vi "LowerLevelSortArrays.vi"(0 "Sorted Array in":string[](array[string]), 1 "DIM-Double-Array":refnum<vi>[](array[refnum]), 2 "DIM-Double":refnum<vi>[](array[refnum]), 3 "DigitalNumeric":refnum<vi>[](array[refnum]), 4 "Boolean":refnum<vi>[](array[refnum]), 5 "DIM-Short":refnum<vi>[](array[refnum]), 6 "Boolean(Strict)":refnum<vi>[](array[refnum]), 7 "Unsorted Array in":string[](array[string]), 8 "Index":i32, 10 "Type":T1(ring)) -> (21 "DIM-Double-Array (sorted)":refnum<vi>[](array[refnum]), 22 "DIM-Double (sorted)":refnum<vi>[](array[refnum]), 23 "DigitalNumeric (sorted)":refnum<vi>[](array[refnum]), 24 "Boolean (sorted)":refnum<vi>[](array[refnum]), 25 "DIM-Short(sorted)":refnum<vi>[](array[refnum]), 26 "Boolean (Strict) (sorted)":refnum<vi>[](array[refnum]), 27 "Sorted Array out":string[](array[string]))   [LabVIEW 2014, in "Panels.lvlib"]
uses:
  Panels.lvlib
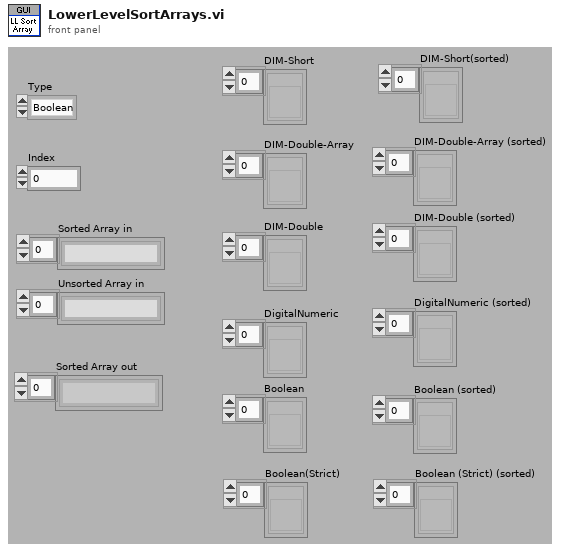
[diagram p1: front panel]
types:
  T1 = enum16{"Boolean", "DigitalNumeric", "DIM-Double", "DIM-Double-Array", "DIM-Short", "Boolean (Strict)"}
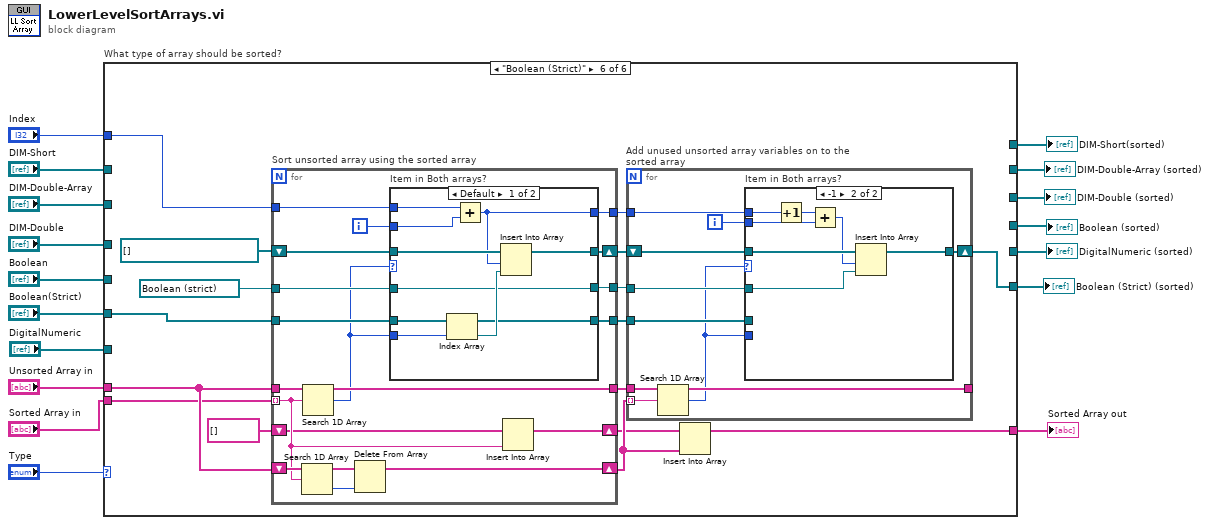
[diagram p0: block diagram]
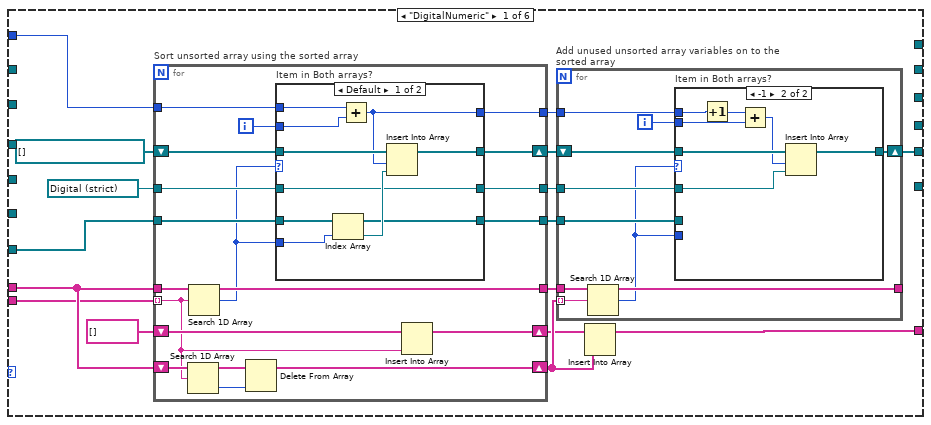
[diagram p2: hidden frame]
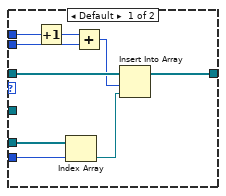
[diagram p3: hidden frame]
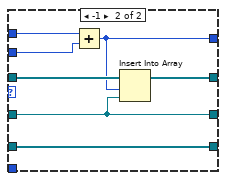
[diagram p4: hidden frame]
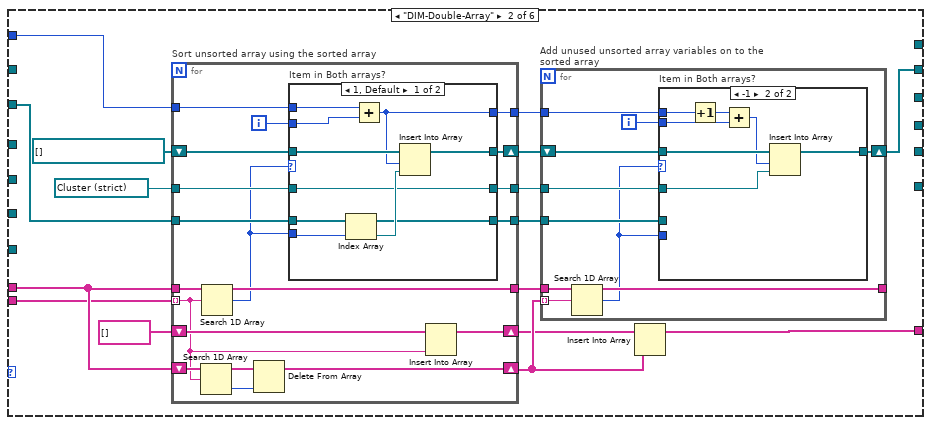
[diagram p5: hidden frame]
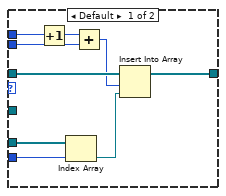
[diagram p6: hidden frame]
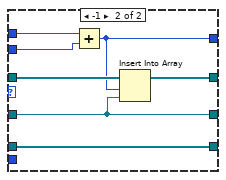
[diagram p7: hidden frame]
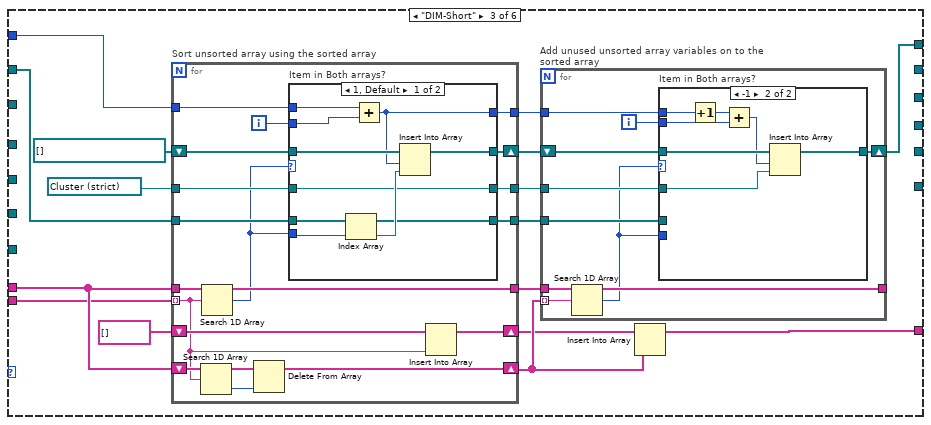
[diagram p8: hidden frame]
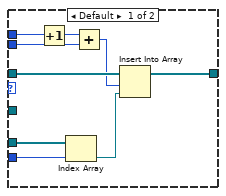
[diagram p9: hidden frame]
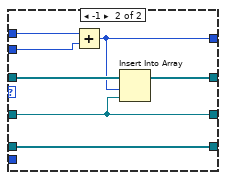
[diagram p10: hidden frame]
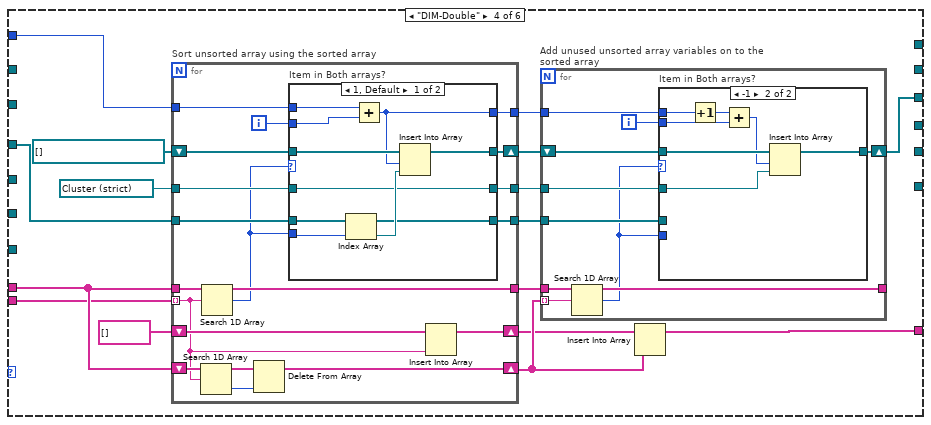
[diagram p11: hidden frame]
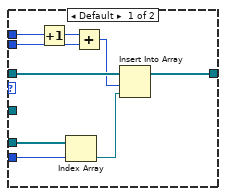
[diagram p12: hidden frame]
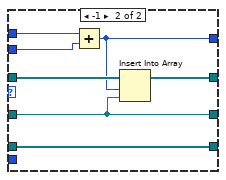
[diagram p13: hidden frame]
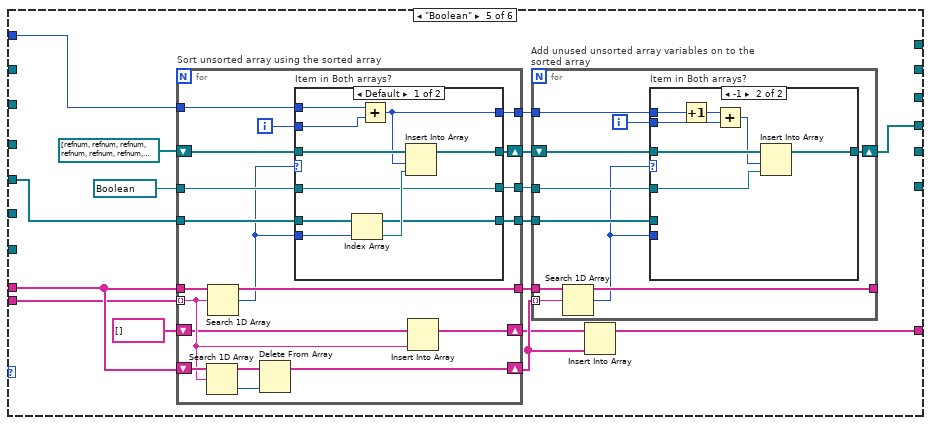
[diagram p14: hidden frame]
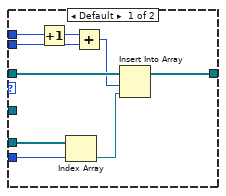
[diagram p15: hidden frame]
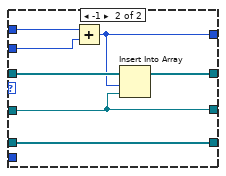
[diagram p16: hidden frame]
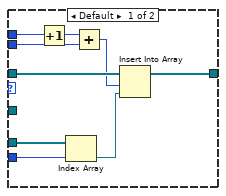
[diagram p17: hidden frame]
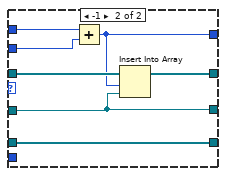
[diagram p18: hidden frame]
diagram:
  n1 = case "What type of array should be sorted?" shown="\"Boolean (Strict)\"" "Type" {
    tunnel: "DigitalNumeric" -> [w32 _ _ _ _ _]
    tunnel: "Unsorted Array in" -> [w31 w105 w179 w250 w324 w400]
    tunnel: "Sorted Array in" -> [w27 w104 w178 w249 w323 w399]
    tunnel: "Index" -> [w30 w107 w181 w255 w329 w403]
    tunnel: "Boolean" -> [_ _ _ _ w326 _]
    tunnel: "DIM-Double" -> [_ _ _ w252 _ _]
    tunnel: [_ _ _ w244 _ _] -> w9
    tunnel: [w28 w106 w180 w251 w325 w401] -> w10
    tunnel: [_ _ _ _ w316 _] -> w8
    tunnel: [w20 _ _ _ _ _] -> w7
    tunnel: "DIM-Double-Array" -> [_ w95 _ _ _ _]
    tunnel: [_ w92 _ _ _ _] -> w5
    tunnel: "DIM-Short" -> [_ _ w169 _ _ _]
    tunnel: [_ _ w168 _ _ _] -> w3
    tunnel: "Boolean(Strict)" -> [_ _ _ _ _ w389]
    tunnel: [_ _ _ _ _ w388] -> w1
    frame "DigitalNumeric" {
      n2 = for "Sort unsorted array using the sorted array" {
        tunnel: w27 -> [w59] mode=indexing
        tunnel: w31 -> [w71]
        tunnel: w32 -> [w72]
        shift-right: [w74] -> w25
        shift-left: refnum<vi>[] [] ("FPIndicator") -> [w75]
        tunnel: [w67] -> w26
        shift-right: [w73] -> w21
        shift-left: w31 -> [w70]
        tunnel: [w71] -> w22
        tunnel: w30 -> [w69]
        tunnel: refnum<vi> refnum ("Q90DefMain_Mon") -> [w66]
        tunnel: [w64] -> w24
        tunnel: [w63] -> w23
        shift-right: [w60] -> w18
        shift-left: string[] [] -> [w61]
        i -> [w68]
        n3 = Search 1D Array(1D array=w70, element=w59) -> (index of element=w65:i32)  [unwired: 1 in]
        n4 = Search 1D Array(1D array=w71, element=w59) -> (index of element=w62:i32)  [unwired: 1 in]
        n5 = Delete From Array(array=w70, index=w65) -> (array with subset deleted=w73:string[])  [unwired: 1 in, 1 out]
        n6 = case "Item in Both arrays?" shown="Default" w62 {
          tunnel: w75 -> [w84 w91]
          tunnel: [w82 w90] -> w74
          tunnel: w72 -> [w76 w85]
          tunnel: w62 -> [w81 _]
          tunnel: w69 -> [w78 w87]
          tunnel: w68 -> [w80 w89]
          tunnel: [w79 w88] -> w67
          tunnel: w66 -> [w77 w86]
          tunnel: [w77 w86] -> w64
          tunnel: [w76 w85] -> w63
          frame Default {
            n7 = Index Array(array=w76, index=w81) -> (element=w83:refnum<vi>)
            n8 = Add(x=w78, y=w80) -> (x+y=w79:i32)
            n9 = Insert Into Array(array=w84, index=w79, new element=w83) -> (w82:refnum<vi>[])
          }
          frame -1 {
            n10 = Add(x=w87, y=w89) -> (x+y=w88:i32)
            n11 = Insert Into Array(array=w91, index=w88, new element=w86) -> (w90:refnum<vi>[])
          }
        }
        n12 = Insert Into Array(array=w61, new element=w59) -> (w60:string[])  [unwired: 1 in]
      }
      n13 = for "Add unused unsorted array variables on to the sorted array" {
        tunnel: w21 -> [w34] mode=indexing
        tunnel: w22 -> [w39]
        tunnel: w23 -> [w40]
        shift-right: [w41] -> w20
        shift-left: w25 -> [w42]
        tunnel: [w39] -> _
        tunnel: w26 -> [w38]
        tunnel: w24 -> [w36]
        i -> [w37]
        n14 = Search 1D Array(1D array=w39, element=w34) -> (index of element=w35:i32)  [unwired: 1 in]
        n15 = case "Item in Both arrays?" shown="-1" w35 {
          tunnel: w42 -> [w51 w58]
          tunnel: [w49 w57] -> w41
          tunnel: w40 -> [w48 _]
          tunnel: w35 -> [w47 _]
          tunnel: w38 -> [w43 w52]
          tunnel: w37 -> [w46 w56]
          tunnel: w36 -> [_ w54]
          frame Default {
            n16 = Increment(x=w43) -> (x+1=w44:i32)
            n17 = Index Array(array=w48, index=w47) -> (element=w50:refnum<vi>)
            n18 = Add(x=w44, y=w46) -> (x+y=w45:i32)
            n19 = Insert Into Array(array=w51, index=w45, new element=w50) -> (w49:refnum<vi>[])
          }
          frame -1 {
            n20 = Increment(x=w52) -> (x+1=w53:i32)
            n21 = Add(x=w53, y=w56) -> (x+y=w55:i32)
            n22 = Insert Into Array(array=w58, index=w55, new element=w54) -> (w57:refnum<vi>[])
          }
        }
      }
      n23 = Insert Into Array(array=w18, new element=w21) -> (w28:string[])  [unwired: 1 in]
    }
    frame "DIM-Double-Array" {
      n24 = for "Sort unsorted array using the sorted array" {
        tunnel: w104 -> [w133] mode=indexing
        tunnel: w105 -> [w145]
        tunnel: w95 -> [w146]
        shift-right: [w148] -> w102
        shift-left: refnum<vi>[] [] ("appended array") -> [w149]
        tunnel: [w140] -> w103
        shift-right: [w147] -> w100
        shift-left: w105 -> [w143]
        tunnel: [w145] -> w101
        tunnel: w107 -> [w142]
        tunnel: refnum<vi> refnum ("GasCellBase_SetData") -> [w139]
        tunnel: [w138] -> w99
        tunnel: [w137] -> w98
        shift-right: [w135] -> w96
        shift-left: string[] [] -> [w134]
        i -> [w141]
        n25 = Search 1D Array(1D array=w143, element=w133) -> (index of element=w144:i32)  [unwired: 1 in]
        n26 = Search 1D Array(1D array=w145, element=w133) -> (index of element=w136:i32)  [unwired: 1 in]
        n27 = Delete From Array(array=w143, index=w144) -> (array with subset deleted=w147:string[])  [unwired: 1 in, 1 out]
        n28 = case "Item in Both arrays?" shown="1, Default" w136 {
          tunnel: w149 -> [w158 w165]
          tunnel: [w156 w164] -> w148
          tunnel: w146 -> [w150 w159]
          tunnel: w136 -> [w155 _]
          tunnel: w142 -> [w152 w161]
          tunnel: w141 -> [w154 w163]
          tunnel: [w153 w162] -> w140
          tunnel: w139 -> [w151 w160]
          tunnel: [w151 w160] -> w138
          tunnel: [w150 w159] -> w137
          frame 1, Default {
            n29 = Index Array(array=w150, index=w155) -> (element=w157:refnum<vi>)
            n30 = Add(x=w152, y=w154) -> (x+y=w153:i32)
            n31 = Insert Into Array(array=w158, index=w153, new element=w157) -> (w156:refnum<vi>[])
          }
          frame -1 {
            n32 = Add(x=w161, y=w163) -> (x+y=w162:i32)
            n33 = Insert Into Array(array=w165, index=w162, new element=w160) -> (w164:refnum<vi>[])
          }
        }
        n34 = Insert Into Array(array=w134, new element=w133) -> (w135:string[])  [unwired: 1 in]
      }
      n35 = for "Add unused unsorted array variables on to the sorted array" {
        tunnel: w100 -> [w108] mode=indexing
        tunnel: w101 -> [w113]
        tunnel: w98 -> [w114]
        shift-right: [w115] -> w92
        shift-left: w102 -> [w116]
        tunnel: [w113] -> _
        tunnel: w103 -> [w112]
        tunnel: w99 -> [w110]
        i -> [w111]
        n36 = Search 1D Array(1D array=w113, element=w108) -> (index of element=w109:i32)  [unwired: 1 in]
        n37 = case "Item in Both arrays?" shown="-1" w109 {
          tunnel: w116 -> [w125 w132]
          tunnel: [w123 w131] -> w115
          tunnel: w114 -> [w122 _]
          tunnel: w109 -> [w121 _]
          tunnel: w112 -> [w117 w126]
          tunnel: w111 -> [w120 w130]
          tunnel: w110 -> [_ w128]
          frame Default {
            n38 = Increment(x=w117) -> (x+1=w118:i32)
            n39 = Index Array(array=w122, index=w121) -> (element=w124:refnum<vi>)
            n40 = Add(x=w118, y=w120) -> (x+y=w119:i32)
            n41 = Insert Into Array(array=w125, index=w119, new element=w124) -> (w123:refnum<vi>[])
          }
          frame -1 {
            n42 = Increment(x=w126) -> (x+1=w127:i32)
            n43 = Add(x=w127, y=w130) -> (x+y=w129:i32)
            n44 = Insert Into Array(array=w132, index=w129, new element=w128) -> (w131:refnum<vi>[])
          }
        }
      }
      n45 = Insert Into Array(array=w96, new element=w100) -> (w106:string[])  [unwired: 1 in]
    }
    frame "DIM-Short" {
      n46 = for "Sort unsorted array using the sorted array" {
        tunnel: w178 -> [w207] mode=indexing
        tunnel: w179 -> [w219]
        tunnel: w169 -> [w220]
        shift-right: [w222] -> w176
        shift-left: refnum<vi>[] [] ("DIM-Short") -> [w223]
        tunnel: [w214] -> w177
        shift-right: [w221] -> w174
        shift-left: w179 -> [w217]
        tunnel: [w219] -> w175
        tunnel: w181 -> [w216]
        tunnel: refnum<vi> refnum ("BOB6FVout_MonData") -> [w213]
        tunnel: [w212] -> w173
        tunnel: [w211] -> w172
        shift-right: [w209] -> w170
        shift-left: string[] [] -> [w208]
        i -> [w215]
        n47 = Search 1D Array(1D array=w217, element=w207) -> (index of element=w218:i32)  [unwired: 1 in]
        n48 = Search 1D Array(1D array=w219, element=w207) -> (index of element=w210:i32)  [unwired: 1 in]
        n49 = Delete From Array(array=w217, index=w218) -> (array with subset deleted=w221:string[])  [unwired: 1 in, 1 out]
        n50 = case "Item in Both arrays?" shown="1, Default" w210 {
          tunnel: w223 -> [w232 w239]
          tunnel: [w230 w238] -> w222
          tunnel: w220 -> [w224 w233]
          tunnel: w210 -> [w229 _]
          tunnel: w216 -> [w226 w235]
          tunnel: w215 -> [w228 w237]
          tunnel: [w227 w236] -> w214
          tunnel: w213 -> [w225 w234]
          tunnel: [w225 w234] -> w212
          tunnel: [w224 w233] -> w211
          frame 1, Default {
            n51 = Index Array(array=w224, index=w229) -> (element=w231:refnum<vi>)
            n52 = Add(x=w226, y=w228) -> (x+y=w227:i32)
            n53 = Insert Into Array(array=w232, index=w227, new element=w231) -> (w230:refnum<vi>[])
          }
          frame -1 {
            n54 = Add(x=w235, y=w237) -> (x+y=w236:i32)
            n55 = Insert Into Array(array=w239, index=w236, new element=w234) -> (w238:refnum<vi>[])
          }
        }
        n56 = Insert Into Array(array=w208, new element=w207) -> (w209:string[])  [unwired: 1 in]
      }
      n57 = for "Add unused unsorted array variables on to the sorted array" {
        tunnel: w174 -> [w182] mode=indexing
        tunnel: w175 -> [w187]
        tunnel: w172 -> [w188]
        shift-right: [w189] -> w168
        shift-left: w176 -> [w190]
        tunnel: [w187] -> _
        tunnel: w177 -> [w186]
        tunnel: w173 -> [w184]
        i -> [w185]
        n58 = Search 1D Array(1D array=w187, element=w182) -> (index of element=w183:i32)  [unwired: 1 in]
        n59 = case "Item in Both arrays?" shown="-1" w183 {
          tunnel: w190 -> [w199 w206]
          tunnel: [w197 w205] -> w189
          tunnel: w188 -> [w196 _]
          tunnel: w183 -> [w195 _]
          tunnel: w186 -> [w191 w200]
          tunnel: w185 -> [w194 w204]
          tunnel: w184 -> [_ w202]
          frame Default {
            n60 = Increment(x=w191) -> (x+1=w192:i32)
            n61 = Index Array(array=w196, index=w195) -> (element=w198:refnum<vi>)
            n62 = Add(x=w192, y=w194) -> (x+y=w193:i32)
            n63 = Insert Into Array(array=w199, index=w193, new element=w198) -> (w197:refnum<vi>[])
          }
          frame -1 {
            n64 = Increment(x=w200) -> (x+1=w201:i32)
            n65 = Add(x=w201, y=w204) -> (x+y=w203:i32)
            n66 = Insert Into Array(array=w206, index=w203, new element=w202) -> (w205:refnum<vi>[])
          }
        }
      }
      n67 = Insert Into Array(array=w170, new element=w174) -> (w180:string[])  [unwired: 1 in]
    }
    frame "DIM-Double" {
      n68 = for "Sort unsorted array using the sorted array" {
        tunnel: w249 -> [w281] mode=indexing
        tunnel: w250 -> [w293]
        tunnel: w252 -> [w294]
        shift-right: [w296] -> w247
        shift-left: refnum<vi>[] [] ("DIMControlMon") -> [w297]
        tunnel: [w288] -> w248
        shift-right: [w295] -> w245
        shift-left: w250 -> [w291]
        tunnel: [w293] -> w246
        tunnel: w255 -> [w290]
        tunnel: refnum<vi> refnum ("Q90DefMain_MonData") -> [w287]
        tunnel: [w286] -> w243
        tunnel: [w285] -> w242
        shift-right: [w283] -> w240
        shift-left: string[] [] -> [w282]
        i -> [w289]
        n69 = Search 1D Array(1D array=w291, element=w281) -> (index of element=w292:i32)  [unwired: 1 in]
        n70 = Search 1D Array(1D array=w293, element=w281) -> (index of element=w284:i32)  [unwired: 1 in]
        n71 = Delete From Array(array=w291, index=w292) -> (array with subset deleted=w295:string[])  [unwired: 1 in, 1 out]
        n72 = case "Item in Both arrays?" shown="1, Default" w284 {
          tunnel: w297 -> [w306 w313]
          tunnel: [w304 w312] -> w296
          tunnel: w294 -> [w298 w307]
          tunnel: w284 -> [w303 _]
          tunnel: w290 -> [w300 w309]
          tunnel: w289 -> [w302 w311]
          tunnel: [w301 w310] -> w288
          tunnel: w287 -> [w299 w308]
          tunnel: [w299 w308] -> w286
          tunnel: [w298 w307] -> w285
          frame 1, Default {
            n73 = Index Array(array=w298, index=w303) -> (element=w305:refnum<vi>)
            n74 = Add(x=w300, y=w302) -> (x+y=w301:i32)
            n75 = Insert Into Array(array=w306, index=w301, new element=w305) -> (w304:refnum<vi>[])
          }
          frame -1 {
            n76 = Add(x=w309, y=w311) -> (x+y=w310:i32)
            n77 = Insert Into Array(array=w313, index=w310, new element=w308) -> (w312:refnum<vi>[])
          }
        }
        n78 = Insert Into Array(array=w282, new element=w281) -> (w283:string[])  [unwired: 1 in]
      }
      n79 = for "Add unused unsorted array variables on to the sorted array" {
        tunnel: w245 -> [w256] mode=indexing
        tunnel: w246 -> [w261]
        tunnel: w242 -> [w262]
        shift-right: [w263] -> w244
        shift-left: w247 -> [w264]
        tunnel: [w261] -> _
        tunnel: w248 -> [w260]
        tunnel: w243 -> [w258]
        i -> [w259]
        n80 = Search 1D Array(1D array=w261, element=w256) -> (index of element=w257:i32)  [unwired: 1 in]
        n81 = case "Item in Both arrays?" shown="-1" w257 {
          tunnel: w264 -> [w273 w280]
          tunnel: [w271 w279] -> w263
          tunnel: w262 -> [w270 _]
          tunnel: w257 -> [w269 _]
          tunnel: w260 -> [w265 w274]
          tunnel: w259 -> [w268 w278]
          tunnel: w258 -> [_ w276]
          frame Default {
            n82 = Increment(x=w265) -> (x+1=w266:i32)
            n83 = Index Array(array=w270, index=w269) -> (element=w272:refnum<vi>)
            n84 = Add(x=w266, y=w268) -> (x+y=w267:i32)
            n85 = Insert Into Array(array=w273, index=w267, new element=w272) -> (w271:refnum<vi>[])
          }
          frame -1 {
            n86 = Increment(x=w274) -> (x+1=w275:i32)
            n87 = Add(x=w275, y=w278) -> (x+y=w277:i32)
            n88 = Insert Into Array(array=w280, index=w277, new element=w276) -> (w279:refnum<vi>[])
          }
        }
      }
      n89 = Insert Into Array(array=w240, new element=w245) -> (w251:string[])  [unwired: 1 in]
    }
    frame "Boolean" {
      n90 = for "Sort unsorted array using the sorted array" {
        tunnel: w323 -> [w357] mode=indexing
        tunnel: w324 -> [w367]
        tunnel: w326 -> [w368]
        shift-right: [w370] -> w319
        shift-left: refnum<vi>[] [refnum, refnum, refnum, refnum, refnum, refnum, refnum, refnum, refnum, refnum, refnum, refnum, refnum, refnum, refnum] ("Pop-up Con.") -> [w371]
        tunnel: [w363] -> w320
        shift-right: [w369] -> w321
        shift-left: w324 -> [w366]
        tunnel: [w367] -> w322
        tunnel: w329 -> [w365]
        tunnel: refnum<vi> refnum ("BOB2DefY") -> [w362]
        tunnel: [w361] -> w318
        tunnel: [w360] -> w317
        shift-right: [w355] -> w315
        shift-left: string[] [] -> [w356]
        i -> [w364]
        n91 = Search 1D Array(1D array=w366, element=w357) -> (index of element=w359:i32)  [unwired: 1 in]
        n92 = Search 1D Array(1D array=w367, element=w357) -> (index of element=w358:i32)  [unwired: 1 in]
        n93 = Delete From Array(array=w366, index=w359) -> (array with subset deleted=w369:string[])  [unwired: 1 in, 1 out]
        n94 = case "Item in Both arrays?" shown="Default" w358 {
          tunnel: w371 -> [w380 w387]
          tunnel: [w378 w386] -> w370
          tunnel: w368 -> [w372 w381]
          tunnel: w358 -> [w377 _]
          tunnel: w365 -> [w374 w383]
          tunnel: w364 -> [w376 w385]
          tunnel: [w375 w384] -> w363
          tunnel: w362 -> [w373 w382]
          tunnel: [w373 w382] -> w361
          tunnel: [w372 w381] -> w360
          frame Default {
            n95 = Index Array(array=w372, index=w377) -> (element=w379:refnum<vi>)
            n96 = Add(x=w374, y=w376) -> (x+y=w375:i32)
            n97 = Insert Into Array(array=w380, index=w375, new element=w379) -> (w378:refnum<vi>[])
          }
          frame -1 {
            n98 = Add(x=w383, y=w385) -> (x+y=w384:i32)
            n99 = Insert Into Array(array=w387, index=w384, new element=w382) -> (w386:refnum<vi>[])
          }
        }
        n100 = Insert Into Array(array=w356, new element=w357) -> (w355:string[])  [unwired: 1 in]
      }
      n101 = for "Add unused unsorted array variables on to the sorted array" {
        tunnel: w321 -> [w330] mode=indexing
        tunnel: w322 -> [w335]
        tunnel: w317 -> [w336]
        shift-right: [w337] -> w316
        shift-left: w319 -> [w338]
        tunnel: [w335] -> _
        tunnel: w320 -> [w334]
        tunnel: w318 -> [w332]
        i -> [w333]
        n102 = Search 1D Array(1D array=w335, element=w330) -> (index of element=w331:i32)  [unwired: 1 in]
        n103 = case "Item in Both arrays?" shown="-1" w331 {
          tunnel: w338 -> [w347 w354]
          tunnel: [w345 w353] -> w337
          tunnel: w336 -> [w344 _]
          tunnel: w331 -> [w343 _]
          tunnel: w334 -> [w339 w348]
          tunnel: w333 -> [w342 w352]
          tunnel: w332 -> [_ w350]
          frame Default {
            n104 = Increment(x=w339) -> (x+1=w340:i32)
            n105 = Index Array(array=w344, index=w343) -> (element=w346:refnum<vi>)
            n106 = Add(x=w340, y=w342) -> (x+y=w341:i32)
            n107 = Insert Into Array(array=w347, index=w341, new element=w346) -> (w345:refnum<vi>[])
          }
          frame -1 {
            n108 = Increment(x=w348) -> (x+1=w349:i32)
            n109 = Add(x=w349, y=w352) -> (x+y=w351:i32)
            n110 = Insert Into Array(array=w354, index=w351, new element=w350) -> (w353:refnum<vi>[])
          }
        }
      }
      n111 = Insert Into Array(array=w315, new element=w321) -> (w325:string[])  [unwired: 1 in]
    }
    frame "Boolean (Strict)" {
      n112 = for "Sort unsorted array using the sorted array" {
        tunnel: w399 -> [w431] mode=indexing
        tunnel: w400 -> [w441]
        tunnel: w389 -> [w442]
        shift-right: [w444] -> w395
        shift-left: refnum<vi>[] [] ("Pop-up Con.") -> [w445]
        tunnel: [w437] -> w396
        shift-right: [w443] -> w397
        shift-left: w400 -> [w440]
        tunnel: [w441] -> w398
        tunnel: w403 -> [w439]
        tunnel: refnum<vi> refnum ("BOB3GVSen") -> [w436]
        tunnel: [w435] -> w394
        tunnel: [w434] -> w393
        shift-right: [w429] -> w392
        shift-left: string[] [] -> [w430]
        i -> [w438]
        n113 = Search 1D Array(1D array=w440, element=w431) -> (index of element=w433:i32)  [unwired: 1 in]
        n114 = Search 1D Array(1D array=w441, element=w431) -> (index of element=w432:i32)  [unwired: 1 in]
        n115 = Delete From Array(array=w440, index=w433) -> (array with subset deleted=w443:string[])  [unwired: 1 in, 1 out]
        n116 = case "Item in Both arrays?" shown="Default" w432 {
          tunnel: w445 -> [w454 w461]
          tunnel: [w452 w460] -> w444
          tunnel: w442 -> [w446 w455]
          tunnel: w432 -> [w451 _]
          tunnel: w439 -> [w448 w457]
          tunnel: w438 -> [w450 w459]
          tunnel: [w449 w458] -> w437
          tunnel: w436 -> [w447 w456]
          tunnel: [w447 w456] -> w435
          tunnel: [w446 w455] -> w434
          frame Default {
            n117 = Index Array(array=w446, index=w451) -> (element=w453:refnum<vi>)
            n118 = Add(x=w448, y=w450) -> (x+y=w449:i32)
            n119 = Insert Into Array(array=w454, index=w449, new element=w453) -> (w452:refnum<vi>[])
          }
          frame -1 {
            n120 = Add(x=w457, y=w459) -> (x+y=w458:i32)
            n121 = Insert Into Array(array=w461, index=w458, new element=w456) -> (w460:refnum<vi>[])
          }
        }
        n122 = Insert Into Array(array=w430, new element=w431) -> (w429:string[])  [unwired: 1 in]
      }
      n123 = for "Add unused unsorted array variables on to the sorted array" {
        tunnel: w397 -> [w404] mode=indexing
        tunnel: w398 -> [w409]
        tunnel: w393 -> [w410]
        shift-right: [w411] -> w388
        shift-left: w395 -> [w412]
        tunnel: [w409] -> _
        tunnel: w396 -> [w408]
        tunnel: w394 -> [w406]
        i -> [w407]
        n124 = Search 1D Array(1D array=w409, element=w404) -> (index of element=w405:i32)  [unwired: 1 in]
        n125 = case "Item in Both arrays?" shown="-1" w405 {
          tunnel: w412 -> [w421 w428]
          tunnel: [w419 w427] -> w411
          tunnel: w410 -> [w418 _]
          tunnel: w405 -> [w417 _]
          tunnel: w408 -> [w413 w422]
          tunnel: w407 -> [w416 w426]
          tunnel: w406 -> [_ w424]
          frame Default {
            n126 = Increment(x=w413) -> (x+1=w414:i32)
            n127 = Index Array(array=w418, index=w417) -> (element=w420:refnum<vi>)
            n128 = Add(x=w414, y=w416) -> (x+y=w415:i32)
            n129 = Insert Into Array(array=w421, index=w415, new element=w420) -> (w419:refnum<vi>[])
          }
          frame -1 {
            n130 = Increment(x=w422) -> (x+1=w423:i32)
            n131 = Add(x=w423, y=w426) -> (x+y=w425:i32)
            n132 = Insert Into Array(array=w428, index=w425, new element=w424) -> (w427:refnum<vi>[])
          }
        }
      }
      n133 = Insert Into Array(array=w392, new element=w397) -> (w401:string[])  [unwired: 1 in]
    }
  }
  "Sorted Array out" <- w10
  "DIM-Double (sorted)" <- w9
  "Boolean (sorted)" <- w8
  "DigitalNumeric (sorted)" <- w7
  "DIM-Double-Array (sorted)" <- w5
  "DIM-Short(sorted)" <- w3
  "Boolean (Strict) (sorted)" <- w1
